vi "7_DvDt_ON.vi"(0 "file path (IN)":path, 1 "TEST #":string, 5 "VCE":dbl, 7 "Project #":string, 9 "Request #":string, 11 "error in (no error)":errorcluster) -> (2 "Dv (V)":dbl, 3 "Dt (ns)":dbl, 4 "file path (OUT)":path, 6 "ON Region":waveform(dbl)[](graph) caption="DvDt on (V/us)", 8 "DONE Dv/Dt ON":bool, 10 "Dv/Dt (V/us)":dbl, 15 "error out":errorcluster)   [LabVIEW 2020]
uses:
  <vilib>/Waveform/WDTOps.llb/WDT Waveform Duration DBL.vi
  <vilib>/Waveform/WDTOps.llb/WDT Get Waveform Subset DBL.vi
  <vilib>/measure/mascope.llb/Transition Measurements 1 chan.vi
  <vilib>/measure/NI_MAPro.lvlib
panel:
  in  "Decision ?":bool
  out "Cursor a : Channel 3":dbl
  out "Cursor b : Channel 3":dbl
  in  "Cursor b : Channel 3\nfall edge number":i32=1 min=1
  in  "Cursor a : Channel 3\nfall edge number":i32=1 min=1
  in  "Cursor b : Channel 3 \nfall edge tolerance":dbl=0.1
  in  "Cursor a : Channel 3 \nfall edge tolerance":dbl=0.1
  out "Dt (us)":dbl
  out "10% Vce":dbl
  out "75% Vce":dbl
  out "measurement info (CH3  Cursor a)":T1 {"ref levels"."ref units" items=["absolute", "relative"]; "ref levels"."high ref level" format="%.2p"; "ref levels"."low ref level" format="%.2p"; "ref levels"."mid ref level" format="%.2p"; "end time" format="%.6e"; "start time" format="%.6e"}
  out "measurement info (CH3 Cursor b)":T1 {"ref levels"."ref units" items=["absolute", "relative"]; "ref levels"."high ref level" format="%.2p"; "ref levels"."low ref level" format="%.2p"; "ref levels"."mid ref level" format="%.2p"; "end time" format="%.6e"; "start time" format="%.6e"}
  in  "reference  levels (CH1 2nd Cursor)":T2={"high ref level"=90.0, "mid ref level"=50.0, "low ref level"=10.0, "ref units"=1} {"ref units" items=["absolute", "percent"]; "high ref level" format="%0.2f"; "low ref level" format="%0.2f"; "mid ref level" format="%0.2f"}
  in  "reference  levels (CH1 1st Cursor)":T2={"high ref level"=90.0, "mid ref level"=50.0, "low ref level"=10.0, "ref units"=1} {"ref units" items=["absolute", "percent"]; "high ref level" format="%0.2f"; "low ref level" format="%0.2f"; "mid ref level" format="%0.2f"}
  out "Waveform Graph":waveform(dbl)[](graph)
  # "From 75% to 10% of Nominal Voltage"
  # "Default = 1"
  # "Default = 1"
  # "Default = 0.1"
  # "Default = 0.1"
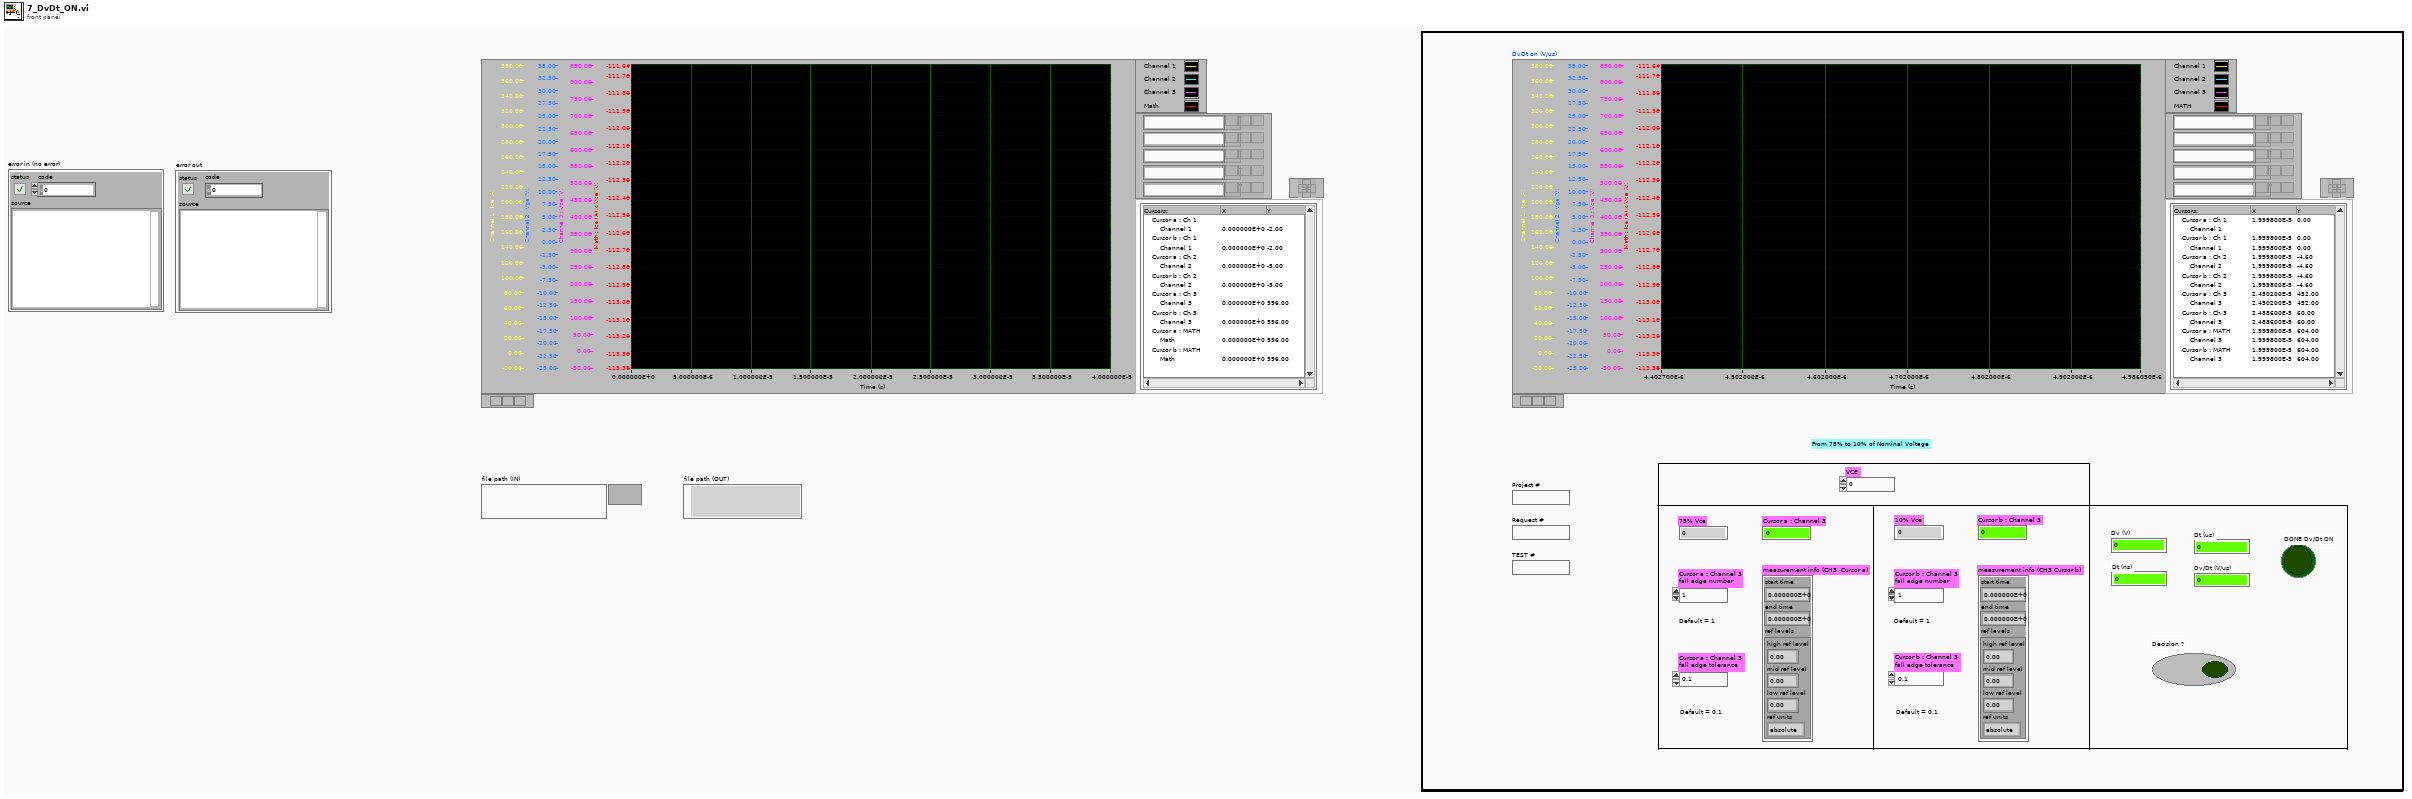
[diagram p1: front panel]
types:
  T1 = cluster{"start time":dbl, "end time":dbl, "ref levels":cluster{"high ref level":dbl, "mid ref level":dbl, "low ref level":dbl, "ref units":u16}}
  T2 = cluster{"high ref level":dbl, "mid ref level":dbl, "low ref level":dbl, "ref units":u16}
  T3 = enum32{"Invalid", "Standard", "Closed", "Hidden", "Minimized", "Maximized"}
  T4 = typedef "imagedata.ctl" = cluster{"image type":i32, "image depth":i32, "image":u8[], "mask":u8[], "colors":u32[], "Rectangle":cluster{"left":i16, "top":i16, "right":i16, "bottom":i16}}
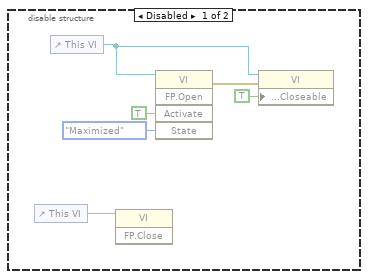
[diagram p2: hidden frame]
diagram:
  w12 = 0.0 ("Dv (V)")
  w13 = errorcluster {"status"=FALSE, "code"=0, "source"=""} ("error out")
  w5 = FALSE ("DONE Tdon")
  w14 = waveform(dbl)[] [] ("Waveform Graph")
  n1 = local write "Cursor a : Channel 3\nfall edge number"(1 ("Cursor a : Channel 3\nfall edge number")) -> ()
  n2 = local write "Cursor a : Channel 3 \nfall edge tolerance"(0.1 ("Cursor a : Channel 3 \nfall edge tolerance")) -> ()
  n3 = local write "Cursor b : Channel 3\nfall edge number"(1 ("Cursor b : Channel 3\nfall edge number")) -> ()
  n4 = local write "Cursor b : Channel 3 \nfall edge tolerance"(0.1 ("Cursor b : Channel 3 \nfall edge tolerance")) -> ()
  n5 = local write "Cursor a : Channel 3"(w12) -> ()
  n6 = local write "Dv (V)"(w12) -> ()
  n7 = local write "Dt (ns)"(w12) -> ()
  n8 = local write "Dt (us)"(w12) -> ()
  n9 = local write "Dv/Dt (V/us)"(w12) -> ()
  n10 = local write "Cursor b : Channel 3"(w12) -> ()
  n11 = local write "error out"(w13) -> ()
  n12 = local write "error in (no error)"(w13) -> ()
  n13 = local write "DONE Dv/Dt ON"(w5) -> ()
  n14 = local write "Waveform Graph"(w14) -> ()
  n15 = local write "ON Region"(w14) -> ()
  n16 = local write "Decision ?"(w5) -> ()
  n17 = disable-structure shown="Enabled" {
    frame Disabled {
      n18 = control-ref of="This VI"() -> (w15:refnum<vi>)
      n19 = control-ref of="This VI"() -> (w16:refnum<vi>)
      n20 = invoke class="VI" method="FP.Close"(reference=w15) -> ()  [unwired: 2 in, 3 out]
      n21 = invoke class="VI" method="FP.Open"(reference=w16, "Activate"=TRUE ("Activate?"), "State"=T3."Maximized") -> (error in=w19:errorcluster, error out=w17:errorcluster)  [unwired: 1 in, 4 out]
      n22 = property class="VI"(reference=w16, error in=w17, "Front Panel.Closeable"=TRUE ("Front Panel Window:Closeable")) -> ()  [unwired: 2 out]
    }
    frame Enabled {
    }
  }
  n23 = flat-sequence {
    tunnel: [w23] -> w7
    tunnel: ["file path (IN)"] -> w6
    tunnel: [w33] -> w11
    tunnel: [w32] -> w8
    tunnel: w7 -> [w31]
    tunnel: w6 -> [w30]
    tunnel: w11 -> [w264]
    tunnel: [w263] -> w10
    tunnel: [w262] -> w9
    tunnel: w8 -> [w262]
    tunnel: w10 -> [w277]
    tunnel: w9 -> [w278]
    frame #0 {
      n24 = control-ref of="This VI"() -> (w28:refnum<vi>)
      n25 = invoke class="VI" method="FP.Open"(reference=w28, error in="error in (no error)", "Activate"=TRUE ("Activate?"), "State"=T3."Maximized") -> (error out=w29:errorcluster)  [unwired: 1 in, 4 out]
      n26 = property class="VI"(reference=w28, error in=w29, "Front Panel.Closeable"=TRUE ("Front Panel Window:Closeable")) -> (error out=w23:errorcluster)  [unwired: 1 out]
    }
    frame #1 {
      n27 = while {
        tunnel: [w38] -> w32
        shift-right: [w39] -> w33
        shift-left: w31 -> [w37]
        tunnel: w30 -> [w35]
        stop <- w41 stop-if-true
        n28 = flat-sequence {
          tunnel: w37 -> [w71]
          tunnel: [w71] -> w36
          tunnel: w35 -> [w70]
          tunnel: [w70] -> w34
          tunnel: [w86] -> w59
          tunnel: [w76] -> w58
          tunnel: [w72] -> w57
          tunnel: w36 -> [w163]
          tunnel: w34 -> [w157]
          tunnel: w59 -> [w206]
          tunnel: [w187] -> w56
          tunnel: w58 -> [w199]
          tunnel: [w199] -> w55
          tunnel: [w186] -> w54
          tunnel: [w185] -> w53
          tunnel: [w184] -> w52
          tunnel: [w183] -> w51
          tunnel: w57 -> [w182]
          tunnel: w56 -> [w234]
          tunnel: [w233] -> w50
          tunnel: w55 -> [w237]
          tunnel: [w237] -> w49
          tunnel: w54 -> [w236]
          tunnel: [w236] -> w48
          tunnel: w53 -> [w235]
          tunnel: [w235] -> w47
          tunnel: w52 -> [w227]
          tunnel: [w227] -> w46
          tunnel: w51 -> [w228]
          tunnel: [w228] -> w45
          tunnel: w50 -> [w238]
          tunnel: w49 -> [w251]
          tunnel: [w251] -> w44
          tunnel: w48 -> [w245]
          tunnel: w47 -> [w246]
          tunnel: w46 -> [w244]
          tunnel: w45 -> [w243]
          tunnel: [w238] -> w43
          tunnel: w44 -> [w256]
          tunnel: w43 -> [w258]
          tunnel: [w257] -> w42
          tunnel: [w256] -> w38
          frame #0 {
            w68 = 0.0 ("Dv (V)")
            w66 = FALSE ("DONE Tdon")
            w69 = waveform(dbl)[] [] ("Waveform Graph")
            n29 = Wait (ms)(milliseconds to wait=u32 200) -> ()  [unwired: 1 out]
            n30 = local write "Cursor a : Channel 3"(w68) -> ()
            n31 = local write "Dv (V)"(w68) -> ()
            n32 = local write "Dt (ns)"(w68) -> ()
            n33 = local write "Dt (us)"(w68) -> ()
            n34 = local write "Dv/Dt (V/us)"(w68) -> ()
            n35 = local write "Cursor b : Channel 3"(w68) -> ()
            n36 = local write "DONE Dv/Dt ON"(w66) -> ()
            n37 = local write "Decision ?"(w66) -> ()
            n38 = local write "Waveform Graph"(w69) -> ()
            n39 = local write "ON Region"(w69) -> ()
          }
          frame #1 {
            w138 = u16 1 items=["Samples", "Relative Time"] ("start/duration format")
            w149 = u16 1 items=["Samples", "Relative Time"] ("start/duration format")
            w150 = u16 1 items=["Samples", "Relative Time"] ("start/duration format")
            # "Channel 1"
            # "Channel 3"
            # "Channel 2"
            # "dt"
            # "Ch2"
            # "Ch1"
            n40 = call "3_ReadDatatoWaveform.vi"("error in (no error)"=w163, "file path (IN)"=w157) -> ("error out"=w132:errorcluster, "Waveform Graph"=→"Waveform Graph":waveform(dbl)[], "file path (OUT)"=w76:path, "dt"=w158:dbl, "Ch 2 Data"=w155:dbl[], "Ch 3 Data"=w159:dbl[], "Ch 1 Data"=w156:dbl[])  [unwired: 3 in]
            n41 = To Time Stamp(1:0.0 ("number")) -> (0:w160:timestamp)
            n42 = disable-structure shown="Enabled" {
              disable-tunnel: w160 -> [w167 _]
              disable-tunnel: w158 -> [w166 _]
              disable-tunnel: w156 -> [w165 _]
              disable-tunnel: [w164 _] -> w137
              frame Enabled {
                # "Channel 1"
                n43 = Bundle By Name("Y"=w165, "dt"=w166, "t0"=w167) -> (w164:waveform(dbl))  [unwired: 1 in]
              }
              frame Disabled {
              }
            }
            n44 = disable-structure shown="Enabled" {
              disable-tunnel: w160 -> [w171 _]
              disable-tunnel: w158 -> [w170 _]
              disable-tunnel: w155 -> [w169 _]
              disable-tunnel: [w168 _] -> w136
              frame Enabled {
                # "Channel 2"
                n45 = Bundle By Name("Y"=w169, "dt"=w170, "t0"=w171) -> (w168:waveform(dbl))  [unwired: 1 in]
              }
              frame Disabled {
              }
            }
            n46 = disable-structure shown="Enabled" {
              disable-tunnel: w160 -> [w175 _]
              disable-tunnel: w158 -> [w174 _]
              disable-tunnel: w159 -> [w173 _]
              disable-tunnel: [w172 _] -> w135
              frame Enabled {
                # "Channel 3"
                n47 = Bundle By Name("Y"=w173, "dt"=w174, "t0"=w175) -> (w172:waveform(dbl))  [unwired: 1 in]
              }
              frame Disabled {
              }
            }
            n48 = call-poly <vilib>:"Waveform Duration.vi"("error in (no error)"=w132, "waveform in"=w135) -> ("error out"=w143:errorcluster, "duration"=w140:dbl, "waveform out"=w142:waveform(dbl))  [unwired: 7 in]
            n49 = call-poly <vilib>:"Waveform Duration.vi"("error in (no error)"=w132, "waveform in"=w136) -> ("error out"=w144:errorcluster, "duration"=w147:dbl, "waveform out"=w145:waveform(dbl))  [unwired: 7 in]
            n50 = call-poly <vilib>:"Waveform Duration.vi"("error in (no error)"=w132, "waveform in"=w137) -> ("error out"=w154:errorcluster, "duration"=w151:dbl, "waveform out"=w153:waveform(dbl))  [unwired: 7 in]
            n51 = Divide(x=w140, y=2.0) -> (x/y=w139:dbl)
            n52 = Divide(x=w147, y=2.0) -> (x/y=w148:dbl)
            n53 = Divide(x=w151, y=2.0) -> (x/y=w133:dbl)
            n54 = call-poly <vilib>:"Get Waveform Subset.vi"("start/duration format"=w138, "error in (no error)"=w143, "duration"=w139, "start samples/time"=w139, "waveform in"=w142) -> ("error out"=w129:errorcluster, "waveform out"=w72:waveform(dbl))  [unwired: 1 in, 2 out]
            n55 = call-poly <vilib>:"Get Waveform Subset.vi"("start/duration format"=w149, "error in (no error)"=w144, "duration"=w148, "start samples/time"=w148, "waveform in"=w145) -> ("error out"=w130:errorcluster, "waveform out"=w88:waveform(dbl))  [unwired: 1 in, 2 out]
            n56 = call-poly <vilib>:"Get Waveform Subset.vi"("start/duration format"=w150, "error in (no error)"=w154, "duration"=w133, "start samples/time"=w133, "waveform in"=w153) -> ("error out"=w131:errorcluster, "waveform out"=w87:waveform(dbl))  [unwired: 1 in, 2 out]
            n57 = Build Array(w87, w88, w72) -> (→"ON Region":waveform(dbl)[])
            n58 = Merge Errors(w131, w130, w129) -> (w84:errorcluster)
            n59 = property on="ON Region" class="WFGraph (strict)"(error in=w84) -> (error out=w83:errorcluster, "Width"=w82:u32)  [unwired: 1 in, 1 out]
            n60 = property on="ON Region" class="WFGraph (strict)"(error in=w83, "Caption.Justify"=enum16{"Left", "Center", "Right"}."Left" ("Caption.Justification"), "Caption.Width"=w82, "Caption.FontBold"=TRUE ("Caption.Font:Bold"), "Caption.FontColor"=u32 16860 ("Caption.Font:Color"), "Caption.FontSize"=u32 24 ("Caption.Font:Size"), "Caption.Text"="DvDt on (V/us)") -> (error out=w78:errorcluster)  [unwired: 1 in, 1 out]
            n61 = property on="ON Region" class="WFGraph (strict)"(error in=w78, "XScale.Offset"=w133) -> (error out=w112:errorcluster)  [unwired: 1 in, 1 out]
            n62 = property on="ON Region" class="WFGraph (strict)"(error in=w112, "Active Cursor"=u32 0, "Cursor.Cursor X"=0.0 ("Cursor.Cursor Position:Cursor X"), "Cursor.Cursor Y"=0.0 ("Cursor.Cursor Position:Cursor Y"), "Cursor.Visible"=FALSE) -> (error out=w111:errorcluster)  [unwired: 1 in, 1 out]
            n63 = property on="ON Region" class="WFGraph (strict)"(error in=w111, "Active Cursor"=u32 1, "Cursor.Cursor X"=0.0 ("Cursor.Cursor Position:Cursor X"), "Cursor.Cursor Y"=0.0 ("Cursor.Cursor Position:Cursor Y"), "Cursor.Visible"=FALSE) -> (error out=w110:errorcluster)  [unwired: 1 in, 1 out]
            n64 = property on="ON Region" class="WFGraph (strict)"(error in=w110, "Active Cursor"=u32 2, "Cursor.Cursor X"=0.0 ("Cursor.Cursor Position:Cursor X"), "Cursor.Cursor Y"=0.0 ("Cursor.Cursor Position:Cursor Y"), "Cursor.Visible"=FALSE) -> (error out=w109:errorcluster)  [unwired: 1 in, 1 out]
            n65 = property on="ON Region" class="WFGraph (strict)"(error in=w109, "Active Cursor"=u32 3, "Cursor.Cursor X"=0.0 ("Cursor.Cursor Position:Cursor X"), "Cursor.Cursor Y"=0.0 ("Cursor.Cursor Position:Cursor Y"), "Cursor.Visible"=FALSE) -> (error out=w92:errorcluster)  [unwired: 1 in, 1 out]
            n66 = property on="ON Region" class="WFGraph (strict)"(error in=w92, "Active Cursor"=u32 4, "Cursor.Cursor X"=0.0 ("Cursor.Cursor Position:Cursor X"), "Cursor.Cursor Y"=0.0 ("Cursor.Cursor Position:Cursor Y"), "Cursor.Visible"=FALSE) -> (error out=w91:errorcluster)  [unwired: 1 in, 1 out]
            n67 = property on="ON Region" class="WFGraph (strict)"(error in=w91, "Active Cursor"=u32 5, "Cursor.Cursor X"=0.0 ("Cursor.Cursor Position:Cursor X"), "Cursor.Cursor Y"=0.0 ("Cursor.Cursor Position:Cursor Y"), "Cursor.Visible"=FALSE) -> (error out=w90:errorcluster)  [unwired: 1 in, 1 out]
            n68 = property on="ON Region" class="WFGraph (strict)"(error in=w90, "Active Cursor"=u32 6, "Cursor.Cursor X"=0.0 ("Cursor.Cursor Position:Cursor X"), "Cursor.Cursor Y"=0.0 ("Cursor.Cursor Position:Cursor Y"), "Cursor.Visible"=FALSE) -> (error out=w89:errorcluster)  [unwired: 1 in, 1 out]
            n69 = property on="ON Region" class="WFGraph (strict)"(error in=w89, "Active Cursor"=u32 7, "Cursor.Cursor X"=0.0 ("Cursor.Cursor Position:Cursor X"), "Cursor.Cursor Y"=0.0 ("Cursor.Cursor Position:Cursor Y"), "Cursor.Visible"=FALSE) -> (error out=w86:errorcluster)  [unwired: 1 in, 1 out]
            n70 = call <vilib>:"Beep.vi"("use system alert? (T)"=FALSE, "duration (msec)"=u32 200, "frequency (Hz)"=u32 2000) -> ()  [unwired: 9 in]
          }
          frame #2 {
            w219 = u16 0 items=["falling", "rising"] ("polarity (rising)")
            w220 = u16 0 items=["falling", "rising"] ("polarity (rising)")
            # "YPOS"
            # "XPOS"
            # "Cursor a : Channel 3"
            # "Cursor b : Channel 3"
            # "Cursor b : Channel 3"
            # "Cursor a : Channel 3"
            # "Cursor b : Channel 3"
            # "Cursor a : Channel 3"
            # "Cursor b : Channel 3"
            # "Cursor a : Channel 3"
            # "End Time 1st Cursor"
            # "End Time 2nd Cursor"
            # "1st PARAMETER : 75% Vce"
            # "Channel 1"
            # "2nd PARAMETER : 10% Vce"
            # "Channel 1"
            n71 = Divide(x=75.0, y=100.0) -> (x/y=w226:dbl)
            n72 = Multiply(x=w226, y="VCE") -> (x*y=w194:dbl)
            "75% Vce" <- w194
            n73 = Add(x=w194, y="Cursor a : Channel 3 \nfall edge tolerance") -> (x+y=w212:dbl)
            n74 = Subtract(x=w194, y="Cursor a : Channel 3 \nfall edge tolerance") -> (x-y=w211:dbl)
            n75 = Bundle By Name(cluster="reference  levels (CH1 1st Cursor)", "high ref level"=w212, "mid ref level"=w194, "low ref level"=w211, "ref units"=u16 0) -> (w208:T2)
            n76 = call-poly <vilib>:"Transition Measurements.vi"("edge number (1)"="Cursor a : Channel 3\nfall edge number", "error in (no error)"=w206, "reference levels"=w208, "polarity (rising)"=w220, "signal in"=w182) -> ("error out"=w203:errorcluster, "measurement info"=w207:T1)  [unwired: 1 in, 4 out]
            "measurement info (CH3  Cursor a)" <- w207
            n77 = Unbundle By Name(w207) -> ("end time"=w183:dbl)
            n78 = property on="ON Region" class="WFGraph (strict)"(error in=w203, "Active Cursor"=u32 4, "Cursor.Cursor X"=w183, "Cursor.Visible"=TRUE, "Cursor.Cursor Name Visible"=TRUE) -> (error out=w192:errorcluster)  [unwired: 1 in, 1 out]
            n79 = property on="ON Region" class="WFGraph (strict)"(error in=w192, "Active Cursor"=u32 4) -> (error out=w190:errorcluster, "Cursor.Cursor Y"=w186:dbl)  [unwired: 1 in, 1 out]
            "Cursor a : Channel 3" <- w186
            n80 = Divide(x=10.0, y=100.0) -> (x/y=w223:dbl)
            n81 = Multiply(x=w223, y="VCE") -> (x*y=w195:dbl)
            "10% Vce" <- w195
            n82 = Add(x=w195, y="Cursor b : Channel 3 \nfall edge tolerance") -> (x+y=w218:dbl)
            n83 = Subtract(x=w195, y="Cursor b : Channel 3 \nfall edge tolerance") -> (x-y=w217:dbl)
            n84 = Bundle By Name(cluster="reference  levels (CH1 2nd Cursor)", "high ref level"=w218, "mid ref level"=w195, "low ref level"=w217, "ref units"=u16 0) -> (w214:T2)
            n85 = call-poly <vilib>:"Transition Measurements.vi"("edge number (1)"="Cursor b : Channel 3\nfall edge number", "error in (no error)"=w190, "reference levels"=w214, "polarity (rising)"=w219, "signal in"=w182) -> ("error out"=w200:errorcluster, "measurement info"=w213:T1)  [unwired: 1 in, 4 out]
            "measurement info (CH3 Cursor b)" <- w213
            n86 = Unbundle By Name(w213) -> ("end time"=w184:dbl)
            n87 = property on="ON Region" class="WFGraph (strict)"(error in=w200, "Active Cursor"=u32 5, "Cursor.Cursor X"=w184, "Cursor.Visible"=TRUE, "Cursor.Cursor Name Visible"=TRUE) -> (error out=w188:errorcluster)  [unwired: 1 in, 1 out]
            n88 = call <vilib>:"Beep.vi"("use system alert? (T)"=FALSE, "duration (msec)"=u32 200, "frequency (Hz)"=u32 2000) -> ()  [unwired: 9 in]
            n89 = property on="ON Region" class="WFGraph (strict)"(error in=w188, "Active Cursor"=u32 5) -> (error out=w187:errorcluster, "Cursor.Cursor Y"=w185:dbl)  [unwired: 1 in, 1 out]
            "Cursor b : Channel 3" <- w185
          }
          frame #3 {
            # "2nd Cursor"
            # "1st Cursor"
            n90 = Subtract(x=w228, y=1e-07) -> (x-y=w229:dbl)
            n91 = Add(x=w227, y=1e-07) -> (x+y=w230:dbl)
            n92 = property on="ON Region" class="WFGraph (strict)"(error in=w234, "XScale.Minimum"=w229, "XScale.Maximum"=w230) -> (error out=w233:errorcluster)  [unwired: 1 in, 1 out]
          }
          frame #4 {
            # "us"
            # "ns"
            n93 = Subtract(x=w246, y=w245) -> (x-y=w242:dbl)
            n94 = Subtract(x=w244, y=w243) -> (x-y=w240:dbl)
            n95 = Absolute Value(x=w242) -> (abs(x)=w241:dbl)
            "Dv (V)" <- w241
            n96 = Absolute Value(x=w240) -> (abs(x)=w239:dbl)
            n97 = Multiply(x=w239, y=1000000000.0) -> (x*y=→"Dt (ns)":dbl)
            n98 = Multiply(x=w239, y=1000000.0) -> (x*y=w248:dbl)
            "Dt (us)" <- w248
            n99 = call <vilib>:"Beep.vi"("use system alert? (T)"=FALSE, "duration (msec)"=u32 200, "frequency (Hz)"=u32 2000) -> ()  [unwired: 9 in]
            n100 = Divide(x=w241, y=w248) -> (x/y=→"Dv/Dt (V/us)":dbl)
          }
          frame #5 {
            n101 = while {
              shift-right: [w259] -> w257
              shift-left: w258 -> [w259]
              stop <- "Decision ?" stop-if-true
              n102 = Wait (ms)(milliseconds to wait=u32 100) -> ()  [unwired: 1 out]
            }
          }
        }
        n103 = while {
          tunnel: [w61] -> w41
          shift-right: [w64] -> w39
          shift-left: w42 -> [w65]
          stop <- w63 stop-if-true
          n104 = Wait (ms)(milliseconds to wait=u32 100) -> ()  [unwired: 1 out]
          n105 = call "Display Message to User"("error in (no error)"=w65) -> ("error out"=w64:errorcluster, "NO"=w61:bool)  [unwired: 9 in]
          n106 = Or(x=w61, y=TRUE) -> (x .or. y?=w63:bool)
        }
        n107 = Wait (ms)(milliseconds to wait=u32 100) -> ()  [unwired: 1 out]
      }
    }
    frame #2 {
      w267 = "_"
      n108 = invoke on="ON Region" class="WFGraph (strict)" method="Get Image"(error in=w264) -> (error out=w270:errorcluster, "image data"=w273:T4)  [unwired: 5 in, 4 out]
      n109 = Concatenate Strings("C:\\Inductive_Switching_Project\\IndSw_Image\\" ("string"), "Project #", w267, "Request #", w267, "TEST #", w267, "DvDton" ("string"), ".png" ("string")) -> (w274:string)
      n110 = String To Path(string=w274) -> (path=w272:path)
      n111 = call <vilib>:"Write PNG File.vi"("error in (no error)"=w270, "image data"=w273, "path to PNG file"=w272) -> ("error out"=w263:errorcluster)  [unwired: 7 in, 1 out]
      "DONE Dv/Dt ON" <- TRUE ("DONE Di/Dt ON")
    }
    frame #3 {
      n112 = disable-structure shown="Enabled" {
        disable-tunnel: w277 -> [w279 _]
        frame Enabled {
          n113 = control-ref of="This VI"() -> (w280:refnum<vi>)
          n114 = invoke class="VI" method="FP.Close"(reference=w280, error in=w279) -> ()  [unwired: 1 in, 3 out]
        }
        frame Disabled {
        }
      }
      "error out" <- w277
      "file path (OUT)" <- w278
    }
  }
